vi "AlliGator Manage Phasor Plots Array.vi"(0 "[Raw Phasor Plot] in":T12[](array[typedef]) {"[Decay Metadata]"."# Folds" min=1; "[Decay Metadata]"."ROI Descriptor"."Contours"."Type" items=["No Selection", "Point", "Line", "Rectangle", "Oval", "Polygon", "Freehand Region", "Annulus", "Unused2", "Unused3", "Broken Line", "Freehand Line", "Rotated Rectangle"]}, 1 "Raw Phasor Plot (empty)":T2[](array[typedef]), 2 "Raw Phasor SDV Plot (empty)":T2[](array[typedef]), 3 "Plot Index (-1: Last)":i32=-1, 4 "Raw Phasor (g, s)":T2, 5 "Raw Phasor SDV":T2, 6 "Plot Name":string, 7 "Phasor Index(-1: Last)":i32=-1, 8 "Phasor Frequency":dbl[unit]=160000000.0, 9 "[Raw Phasor Plot] Action":T11, 10 "Calibration Phasor":T1, 11 "Phasor Metadata":T4[](array[typedef]) {"# Folds" min=1; "ROI Descriptor"."Contours"."Type" items=["No Selection", "Point", "Line", "Rectangle", "Oval", "Polygon", "Freehand Region", "Annulus", "Unused2", "Unused3", "Broken Line", "Freehand Line", "Rotated Rectangle"]}, 12 "[Calibration Phasor]":T1[](array[typedef]), 13 "Phasor SDV Options":T3={"Compute Estimated SDV"=FALSE, "# Replicas"=100, "Use Estimated Average Phasor"=FALSE}) -> (14 "[Raw Phasor Plot] out":T12[](array[typedef]) {"[Decay Metadata]"."# Folds" min=1; "[Decay Metadata]"."ROI Descriptor"."Contours"."Type" items=["No Selection", "Point", "Line", "Rectangle", "Oval", "Polygon", "Freehand Region", "Annulus", "Unused2", "Unused3", "Broken Line", "Freehand Line", "Rotated Rectangle"]})   [LabVIEW 2021, in "AlliGator Phasor Graph.lvlib"]
doc: "Handles addition to/deletion from the internal data structure used to store phasor plots and their associated data and metadata."
uses:
  AlliGator Phasor Graph.lvlib
  AlliGator Raw Phasor Plot Data v4.ctl
  Phasor/Phasor (g, s).ctl
  AlliGator Decay Metadata v3.ctl
  Decay Analysis/Decay Preprocessing/AlliGator Decay Background Subtraction Info.ctl
  Decay Analysis/Decay Preprocessing/AlliGator Baseline Subtraction Method.ctl
  Graphs/XY Graph/XY Graph Plot Shift Parameters.ctl
  Graphs/XY Graph/XY Graph Plot Shift Method.ctl
  Decay Analysis/Decay Preprocessing/AlliGator Decay Extrapolation Parameters.ctl
  Phasor/Phasor Standard Deviation Options.ctl
  Phasor/Calibration Phasor (m, phi).ctl
  AlliGator Raw Phasor Plot Array Action.ctl
  Phasor/Phasor.lvlib
  Arrays/Arrays.lvlib
  Decay Analysis/Decay Preprocessing/AlliGator Decay Preprocessing.lvlib
  Graphs/XY Graph/XY Graph Add-Ons.lvlib
panel:
  # "see the AlliGator License on the block diagram (Ctrl+E or Window:Show Block Diagram)"
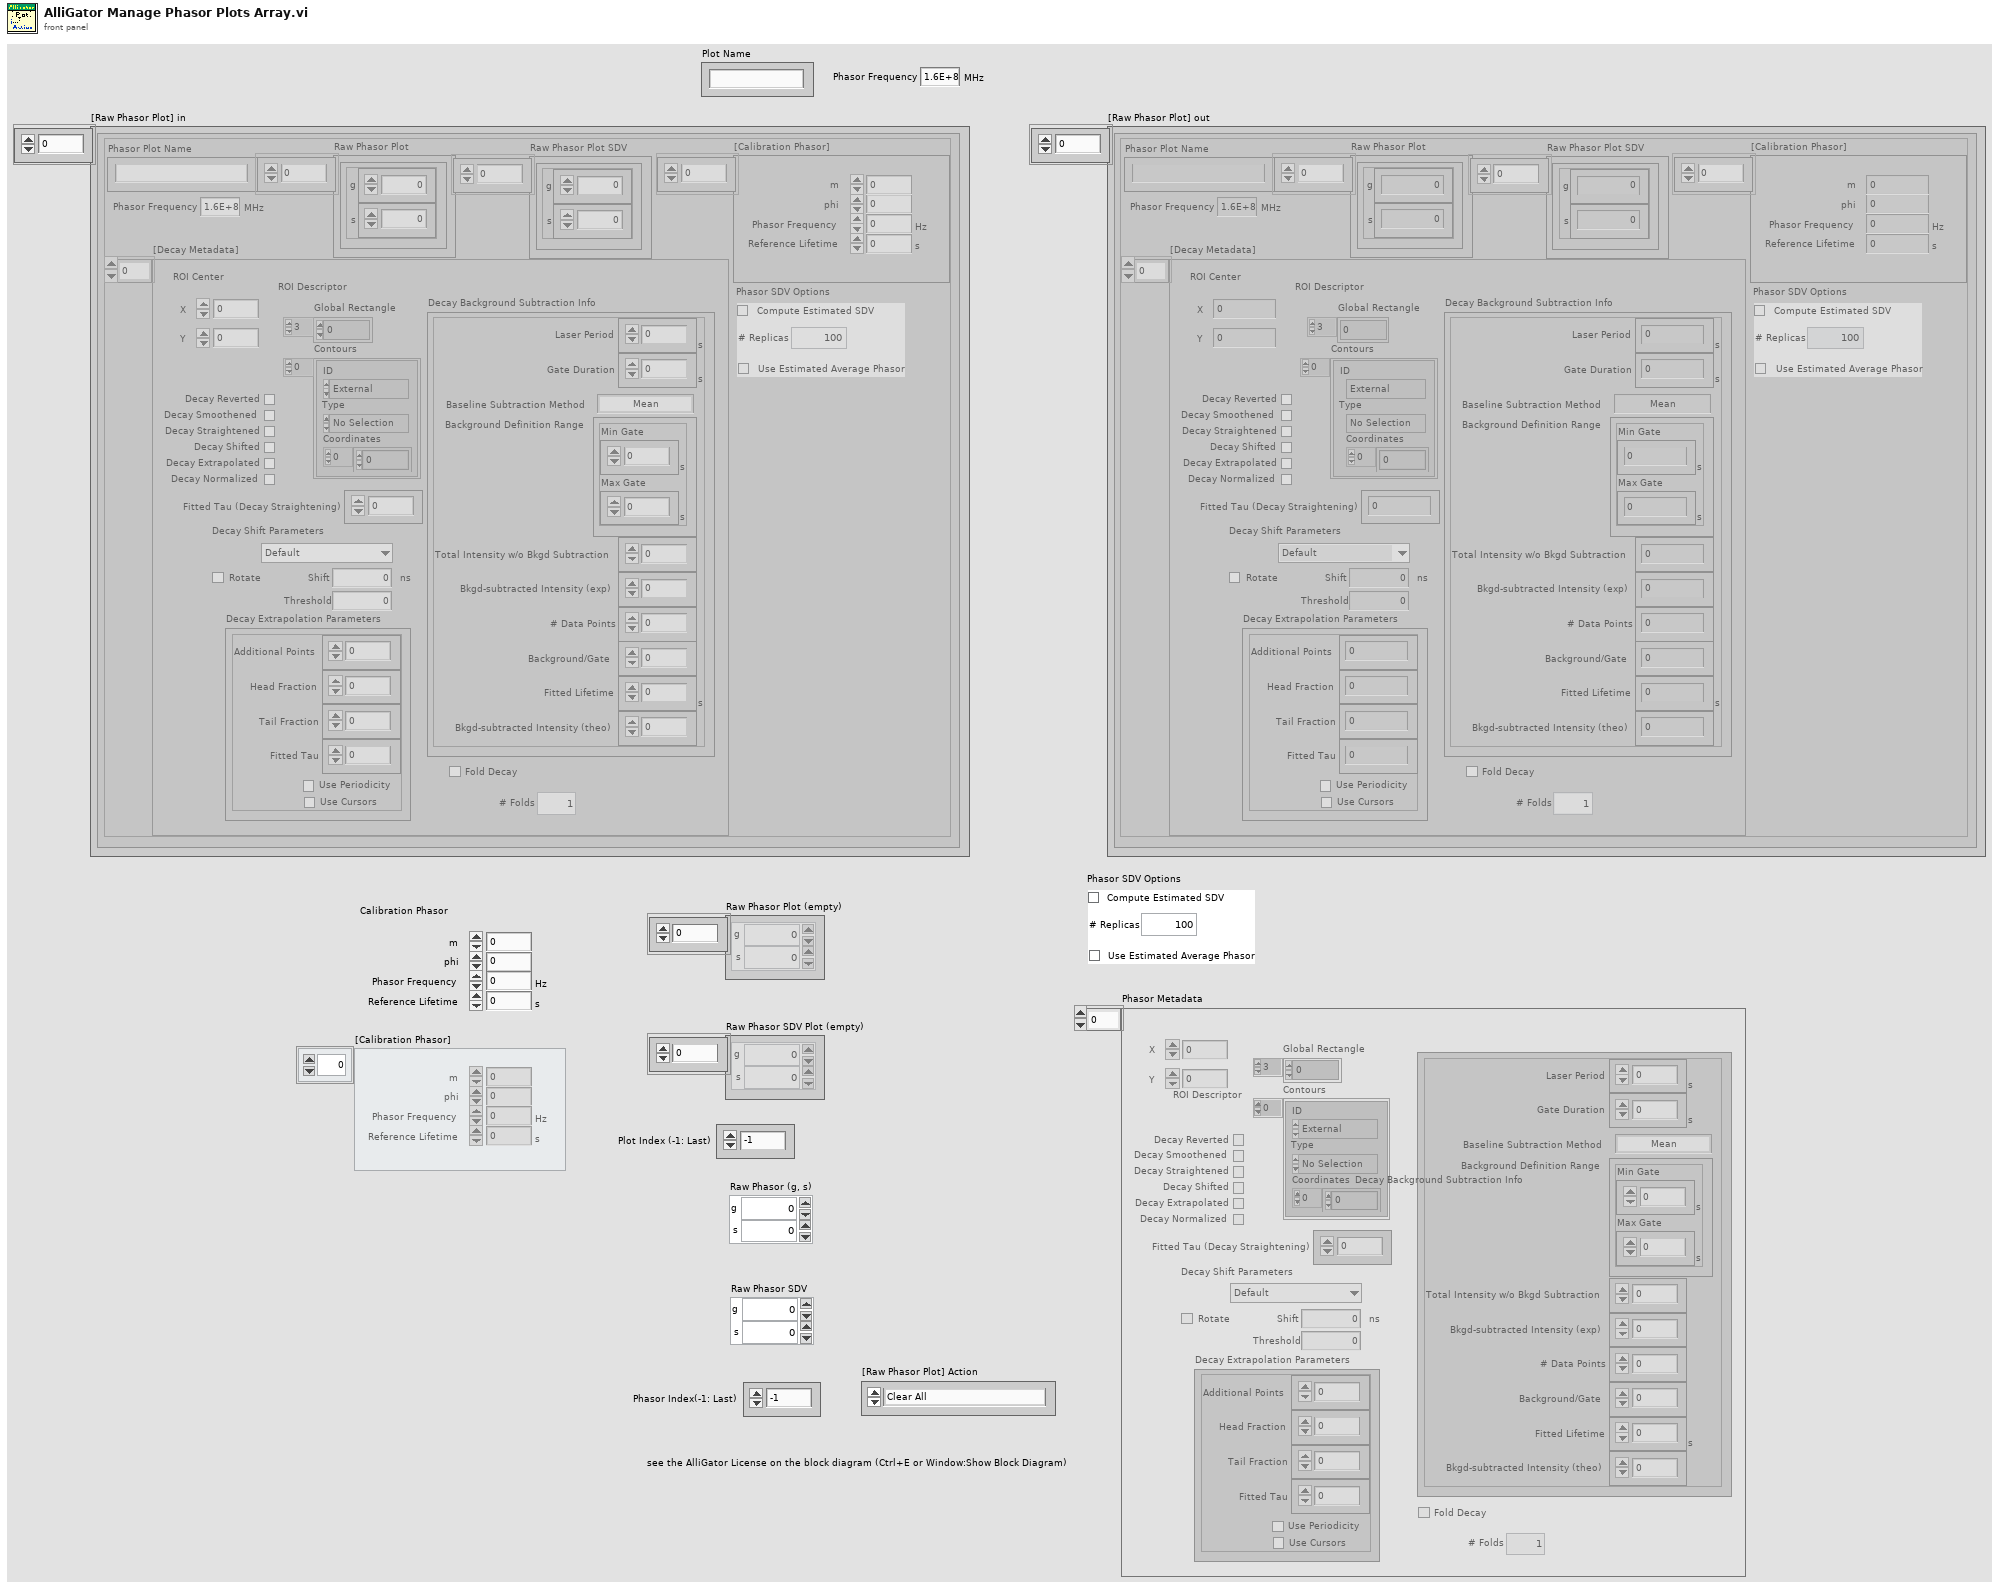
[diagram p1: front panel]
types:
  T1 = typedef "Phasor.lvlib/Calibration Phasor (m, phi).ctl" = cluster{"m":dbl, "phi":dbl, "Phasor Frequency":dbl[unit], "Reference Lifetime":dbl[unit]}
  T2 = typedef "Phasor.lvlib/Phasor (g, s).ctl" = cluster{"g":dbl, "s":dbl}
  T3 = typedef "Phasor.lvlib/Phasor Standard Deviation Options.ctl" = cluster{"Compute Estimated SDV":bool, "# Replicas":u32, "Use Estimated Average Phasor":bool}
  T4 = typedef "AlliGator Phasor Graph.lvlib/AlliGator Decay Metadata v3.ctl" = cluster{"ROI Descriptor":T5, "ROI Center":cluster{"X":i32, "Y":i32}, "Decay Background Subtraction Info":T6, "Decay Reverted":bool, "Decay Smoothened":bool, "Decay Straightened":bool, "Fitted Tau (Decay Straightening)":dbl, "Decay Shift Parameters":T8, "Decay Shifted":bool, "Decay Extrapolated":bool, "Decay Extrapolation Parameters":T10, "Decay Normalized":bool, "Fold Decay":bool, "# Folds":u32}
  T5 = typedef "ROI Descriptor" = cluster{"Global Rectangle":i32[], "Contours":cluster{"ID":enum32{"External", "Internal"}, "Type":u32, "Coordinates":i32[]}[]}
  T6 = typedef "AlliGator Decay Preprocessing.lvlib/AlliGator Decay Background Subtraction Info.ctl" = cluster{"Laser Period":dbl[unit], "Gate Duration":dbl[unit], "Baseline Subtraction Method":T7, "Background Definition Range":cluster{"Min Gate":dbl[unit], "Max Gate":dbl[unit]}, "Total Intensity w/o Bkgd Subtraction":dbl, "Bkgd-subtracted Intensity (exp)":dbl, "# Data Points":i32, "Background/Gate":dbl, "Fitted Lifetime":dbl[unit], "Bkgd-subtracted Intensity (theo)":dbl}
  T7 = typedef "AlliGator Decay Preprocessing.lvlib/AlliGator Baseline Subtraction Method.ctl" = enum16{"Mean", "Min", "Square Gated Single-Exponential", "File", "Constant"}
  T8 = typedef "XY Graph Add-Ons.lvlib/XY Graph Plot Shift Parameters.ctl" = cluster{"Type":T9, "Shift":dbl[unit], "Threshold":dbl, "Rotate":bool}
  T9 = typedef "XY Graph Add-Ons.lvlib/XY Graph Plot Shift Method.ctl" = enum16{"Default", "CFD", "Threshold", "Cross-Correlation"}
  T10 = typedef "AlliGator Decay Preprocessing.lvlib/AlliGator Decay Extrapolation Parameters.ctl" = cluster{"Additional Points":u32, "Head Fraction":dbl, "Fitted Tau":dbl, "Use Periodicity":bool, "Use Cursors":bool, "Tail Fraction":dbl}
  T11 = typedef "AlliGator Phasor Graph.lvlib/AlliGator Raw Phasor Plot Array Action.ctl" = enum16{"Clear All", "-", "Add Raw Phasor Plot", "Delete Raw Phasor Plot", "Replace Raw Phasor Plot", "---------------------", "Add Phasor to Plot", "Replace Phasor in Plot", "Remove Phasor in Plot"}
  T12 = typedef "AlliGator Phasor Graph.lvlib/AlliGator Raw Phasor Plot Data v4.ctl" = cluster{"Phasor Plot Name":string, "Raw Phasor Plot":T2[], "Phasor Frequency":dbl[unit], "[Decay Metadata]":T4[], "Raw Phasor Plot SDV":T2[], "Phasor SDV Options":T3, "[Calibration Phasor]":T1[]}
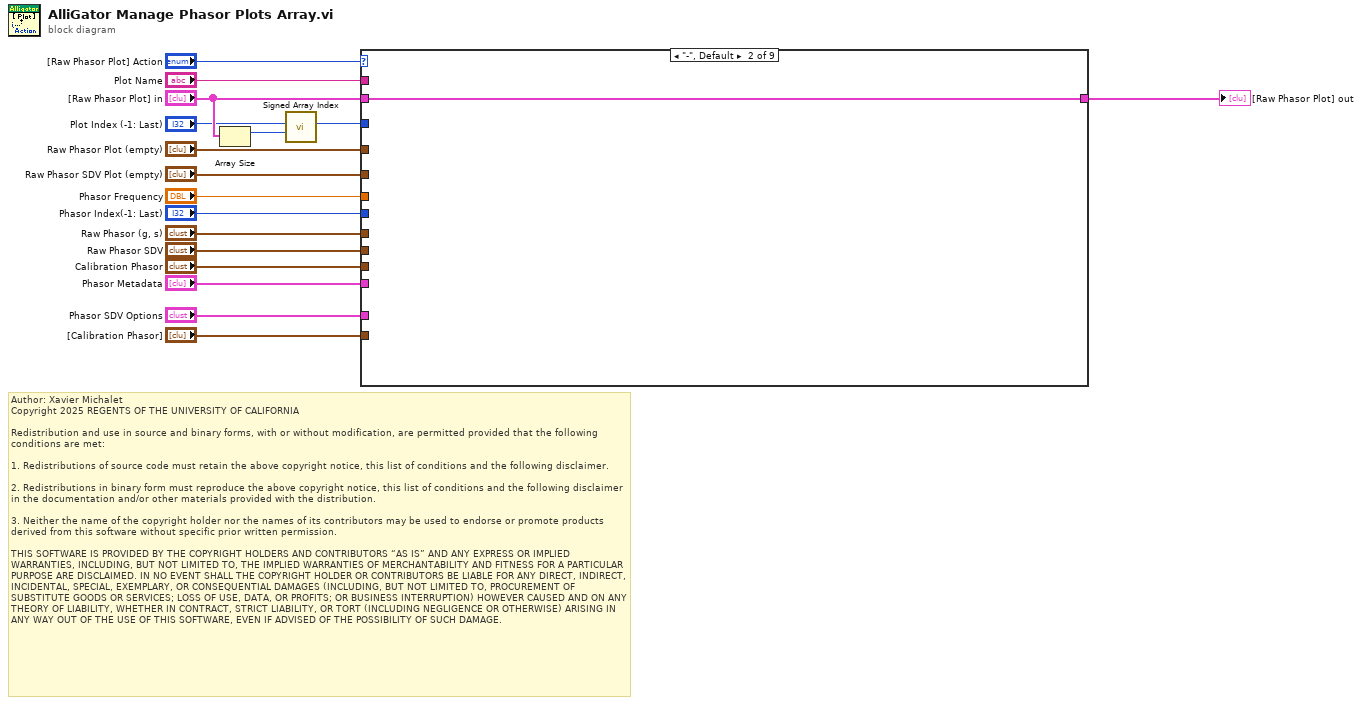
[diagram p0: block diagram]
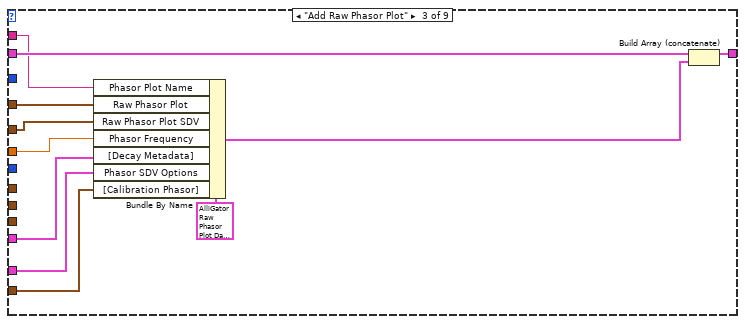
[diagram p3: hidden frame]
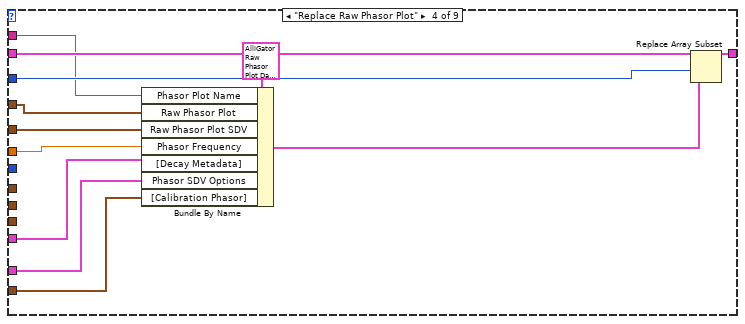
[diagram p4: hidden frame]
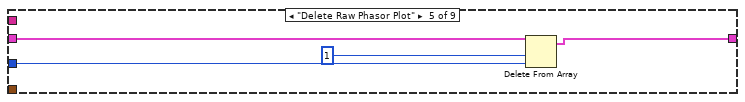
[diagram p5: hidden frame]
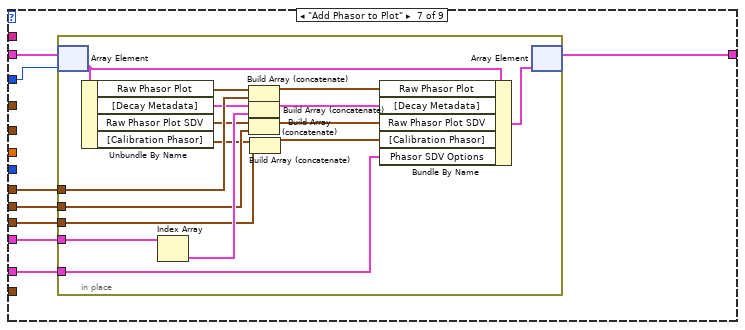
[diagram p7: hidden frame]
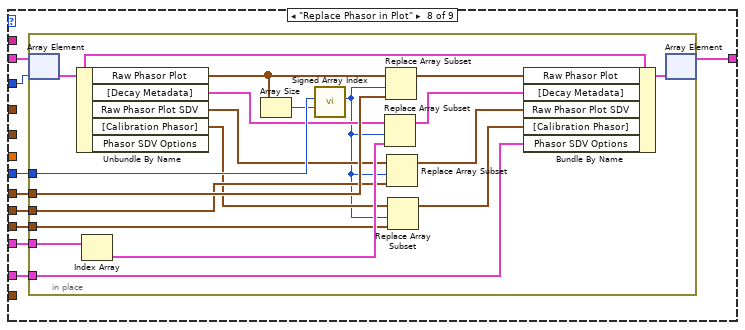
[diagram p8: hidden frame]
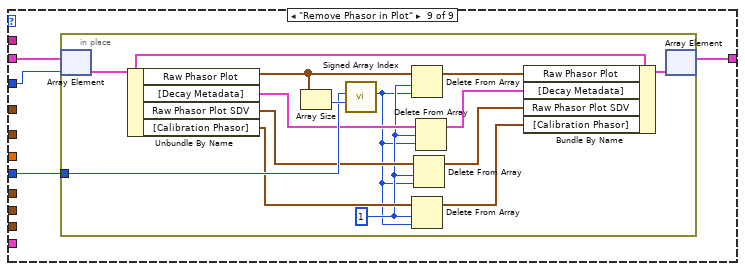
[diagram p9: hidden frame]
diagram:
  # "Author: Xavier Michalet\nCopyright 2025 REGENTS OF THE UNIVERSITY OF CALIFORNIA\n\nRedistribution and use in source and binary forms, with or without modification, are permitted provided that the following conditions are met:\n\n1. Redistributions of source code must retain the above copyright notice, this list of conditions and the following disclaimer.\n\n2. Redistributions in binary form must reproduce the above copyright notice, this list of conditions and the following disclaimer in the documentation and/or other materials provided with the distribution.\n\n3. Neither the name of the copyright holder nor the names of its contributors may be used to endorse or promote products derived from this software without specific prior written permission.\n\nTHIS SOFTWARE IS PROVIDED BY THE COPYRIGHT HOLDERS AND CONTRIBUTORS “AS IS” AND ANY EXPRESS OR IMPLIED WARRANTIES, INCLUDING, BUT NOT LIMITED TO, THE IMPLIED WARRANTIES OF MERCHANTABILITY AND FITNESS FOR A PARTICULAR PURPOSE ARE DISCLAIMED. IN NO EVENT SHALL THE COPYRIGHT HOLDER OR CONTRIBUTORS BE LIABLE FOR ANY DIRECT, INDIRECT, INCIDENTAL, SPECIAL, EXEMPLARY, OR CONSEQUENTIAL DAMAGES (INCLUDING, BUT NOT LIMITED TO, PROCUREMENT OF SUBSTITUTE GOODS OR SERVICES; LOSS OF USE, DATA, OR PROFITS; OR BUSINESS INTERRUPTION) HOWEVER CAUSED AND ON ANY THEORY OF LIABILITY, WHETHER IN CONTRACT, STRICT LIABILITY, OR TORT (INCLUDING NEGLIGENCE OR OTHERWISE) ARISING IN ANY WAY OUT OF THE USE OF THIS SOFTWARE, EVEN IF ADVISED OF THE POSSIBILITY OF SUCH DAMAGE."
  n1 = Array Size(array="[Raw Phasor Plot] in") -> (size(s)=w9:i32)
  n2 = call "Signed Array Index.vi"("Array Size"=w9, "Array Index in"="Plot Index (-1: Last)") -> ("Array Index out"=w10:i32)  [unwired: 9 in]
  n3 = case shown="\"-\", Default" "[Raw Phasor Plot] Action" {
    tunnel: "[Raw Phasor Plot] in" -> [_ w18 w29 w38 w45 w46 w54 w79 w102]
    tunnel: [_ w18 w28 w41 w44 w46 w52 w77 w100] -> w16
    tunnel: w10 -> [_ _ _ w37 w43 _ w53 w78 w101]
    tunnel: "Raw Phasor Plot (empty)" -> [_ _ w25 w40 _ _ _ _ _]
    tunnel: "Raw Phasor (g, s)" -> [_ _ _ _ _ _ w51 w76 _]
    tunnel: "Phasor Index(-1: Last)" -> [_ _ _ _ _ _ _ w75 w99]
    tunnel: "Phasor Frequency" -> [_ _ w22 w36 _ _ _ _ _]
    tunnel: "Plot Name" -> [_ _ w24 w35 _ _ _ _ _]
    tunnel: "Phasor Metadata" -> [_ _ w23 w34 _ _ w50 w74 _]
    tunnel: "Raw Phasor SDV" -> [_ _ _ _ _ _ w49 w72 _]
    tunnel: "Phasor SDV Options" -> [_ _ w20 w31 _ _ w48 w73 _]
    tunnel: "Raw Phasor SDV Plot (empty)" -> [_ _ w21 w32 _ _ _ _ _]
    tunnel: "Calibration Phasor" -> [_ _ _ _ _ _ w47 w71 _]
    tunnel: "[Calibration Phasor]" -> [_ _ w19 w30 _ _ _ _ _]
    frame "Clear All" {
    }
    frame "-", Default {
    }
    frame "Add Raw Phasor Plot" {
      n4 = Bundle By Name(cluster=T12 {"Phasor Plot Name"="", "Raw Phasor Plot"=[], "Phasor Frequency"=160000000.0, "[Decay Metadata]"=[], "Raw Phasor Plot SDV"=[], "Phasor SDV Options"={"Compute Estimated SDV"=FALSE, "# Replicas"=100, "Use Estimated Average Phasor"=FALSE}, "[Calibration Phasor]"=[]} ("array"), "Phasor Plot Name"=w24, "Raw Phasor Plot"=w25, "Raw Phasor Plot SDV"=w21, "Phasor Frequency"=w22, "[Decay Metadata]"=w23, "Phasor SDV Options"=w20, "[Calibration Phasor]"=w19) -> (w27:T12)
      n5 = Build Array (concatenate)(w29, w27) -> (w28:T12[])
    }
    frame "Replace Raw Phasor Plot" {
      n6 = Bundle By Name(cluster=T12 {"Phasor Plot Name"="", "Raw Phasor Plot"=[], "Phasor Frequency"=160000000.0, "[Decay Metadata]"=[], "Raw Phasor Plot SDV"=[], "Phasor SDV Options"={"Compute Estimated SDV"=FALSE, "# Replicas"=100, "Use Estimated Average Phasor"=FALSE}, "[Calibration Phasor]"=[]} ("array"), "Phasor Plot Name"=w35, "Raw Phasor Plot"=w40, "Raw Phasor Plot SDV"=w32, "Phasor Frequency"=w36, "[Decay Metadata]"=w34, "Phasor SDV Options"=w31, "[Calibration Phasor]"=w30) -> (w39:T12)
      n7 = Replace Array Subset(array=w38, new element=w39, index=w37) -> (w41:T12[])
    }
    frame "Delete Raw Phasor Plot" {
      n8 = Delete From Array(array=w45, length=1, index=w43) -> (array with subset deleted=w44:T12[])  [unwired: 1 out]
    }
    frame "---------------------" {
    }
    frame "Add Phasor to Plot" {
      n9 = in-place {
        in-place-border: w51 -> [w67]
        in-place-border: w50 -> [w62]
        in-place-border: w49 -> [w60]
        in-place-border: w48 -> [w58]
        in-place-border: w47 -> [w55]
        n10 = in-place-array #1(w54, w53) -> (w70:T12)
        n11 = Unbundle By Name(w70) -> ("Raw Phasor Plot"=w68:T2[], "[Decay Metadata]"=w65:T4[], "Raw Phasor Plot SDV"=w61:T2[], "[Calibration Phasor]"=w57:T1[])
        n12 = Index Array(array=w62) -> (element=w63:T4)  [unwired: 1 in]
        n13 = Build Array (concatenate)(w68, w67) -> (w66:T2[])
        n14 = Build Array (concatenate)(w65, w63) -> (w64:T4[])
        n15 = Build Array (concatenate)(w61, w60) -> (w59:T2[])
        n16 = Build Array (concatenate)(w57, w55) -> (w56:T1[])
        n17 = Bundle By Name(cluster=w70, "Raw Phasor Plot"=w66, "[Decay Metadata]"=w64, "Raw Phasor Plot SDV"=w59, "[Calibration Phasor]"=w56, "Phasor SDV Options"=w58) -> (w69:T12)
        n18 = in-place-array #1(w69) -> (w52:T12[])  [unwired: 1 out]
      }
    }
    frame "Replace Phasor in Plot" {
      n19 = in-place {
        in-place-border: w76 -> [w95]
        in-place-border: w75 -> [w94]
        in-place-border: w74 -> [w90]
        in-place-border: w73 -> [w87]
        in-place-border: w72 -> [w85]
        in-place-border: w71 -> [w82]
        n20 = in-place-array #2(w79, w78) -> (w98:T12)
        n21 = Unbundle By Name(w98) -> ("Raw Phasor Plot"=w93:T2[], "[Decay Metadata]"=w91:T4[], "Raw Phasor Plot SDV"=w86:T2[], "[Calibration Phasor]"=w83:T1[])  [unwired: 1 out]
        n22 = Index Array(array=w90) -> (element=w89:T4)  [unwired: 1 in]
        n23 = Array Size(array=w93) -> (size(s)=w92:i32)
        n24 = call "Signed Array Index.vi"("Array Size"=w92, "Array Index in"=w94) -> ("Array Index out"=w81:i32)  [unwired: 9 in]
        n25 = Replace Array Subset(array=w91, new element=w89, index=w81) -> (w88:T4[])
        n26 = Replace Array Subset(array=w93, new element=w95, index=w81) -> (w96:T2[])
        n27 = Replace Array Subset(array=w86, new element=w85, index=w81) -> (w84:T2[])
        n28 = Replace Array Subset(array=w83, new element=w82, index=w81) -> (w80:T1[])
        n29 = Bundle By Name(cluster=w98, "Raw Phasor Plot"=w96, "[Decay Metadata]"=w88, "Raw Phasor Plot SDV"=w84, "[Calibration Phasor]"=w80, "Phasor SDV Options"=w87) -> (w97:T12)
        n30 = in-place-array #2(w97) -> (w77:T12[])  [unwired: 1 out]
      }
    }
    frame "Remove Phasor in Plot" {
      n31 = in-place {
        in-place-border: w99 -> [w112]
        w104 = 1 ("length")
        n32 = in-place-array #3(w102, w101) -> (w116:T12)
        n33 = Unbundle By Name(w116) -> ("Raw Phasor Plot"=w111:T2[], "[Decay Metadata]"=w110:T4[], "Raw Phasor Plot SDV"=w108:T2[], "[Calibration Phasor]"=w106:T1[])
        n34 = Array Size(array=w111) -> (size(s)=w113:i32)
        n35 = call "Signed Array Index.vi"("Array Size"=w113, "Array Index in"=w112) -> ("Array Index out"=w103:i32)  [unwired: 9 in]
        n36 = Delete From Array(array=w111, length=w104, index=w103) -> (array with subset deleted=w114:T2[])  [unwired: 1 out]
        n37 = Delete From Array(array=w106, length=w104, index=w103) -> (array with subset deleted=w105:T1[])  [unwired: 1 out]
        n38 = Delete From Array(array=w108, length=w104, index=w103) -> (array with subset deleted=w107:T2[])  [unwired: 1 out]
        n39 = Delete From Array(array=w110, length=w104, index=w103) -> (array with subset deleted=w109:T4[])  [unwired: 1 out]
        n40 = Bundle By Name(cluster=w116, "Raw Phasor Plot"=w114, "[Decay Metadata]"=w109, "Raw Phasor Plot SDV"=w107, "[Calibration Phasor]"=w105) -> (w115:T12)
        n41 = in-place-array #3(w115) -> (w100:T12[])  [unwired: 1 out]
      }
    }
  }
  "[Raw Phasor Plot] out" <- w16
